vi "CCTestProgram.vi"() -> ()   [LabVIEW 2013, in "Medimatic.lvlib"]
uses:
  Medimatic.lvlib
  <userlib>/_MGI/Error Handling/MGI Suppress Error Code/MGI Suppress Error Code (Scalar).vi
  <vilib>/Utility/cursorutil.llb/Set Cursor (Icon Pict).vi
panel:
  out "patientsRetrieved":i32
  out "VerificationSCU":bool=TRUE
  in  "Exit":bool
  in  "queryWorklist":bool
  out "Worklist":string[][](array[string])
  in  "remotePort":i32=1234
  in  "remoteHost":string="localhost"
  in  "remoteAE":string="OFFIS"
  in  "clientAETitle":string="PseudoSCU"
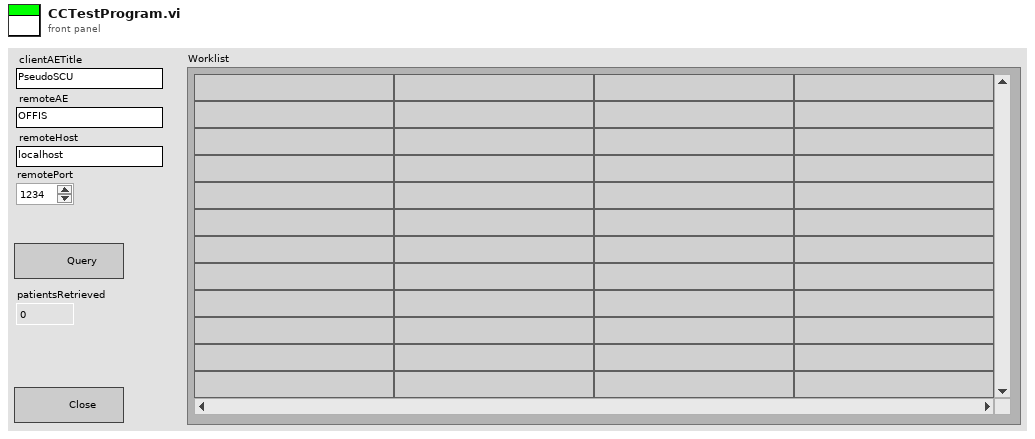
[diagram p1: front panel]
types:
  T1 = typedef "LVPoint32TypeDef.ctl" = cluster{"Horizontal":i32, "Vertical":i32}
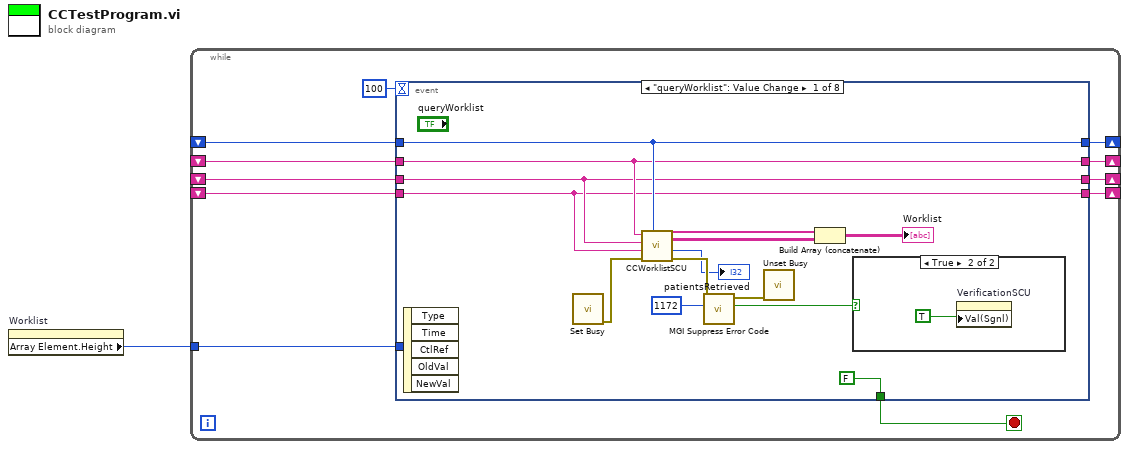
[diagram p0: block diagram]
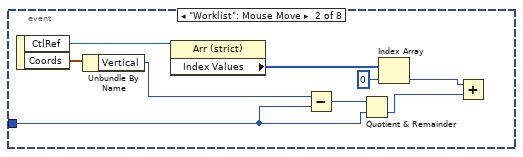
[diagram p3: hidden frame]
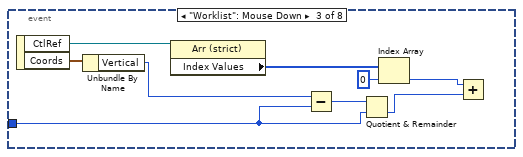
[diagram p4: hidden frame]
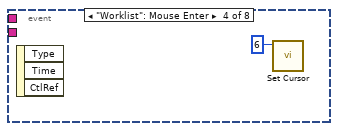
[diagram p5: hidden frame]
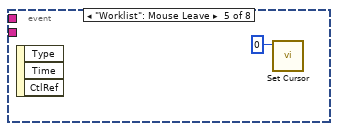
[diagram p6: hidden frame]
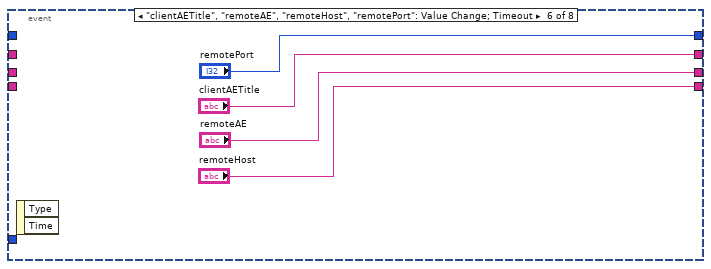
[diagram p7: hidden frame]
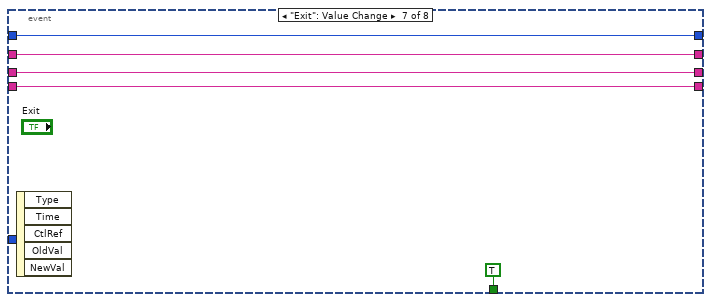
[diagram p8: hidden frame]
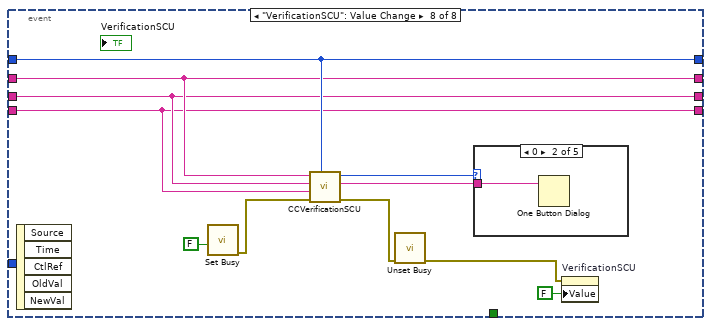
[diagram p9: hidden frame]
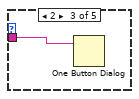
[diagram p11: hidden frame]
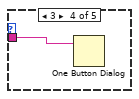
[diagram p12: hidden frame]
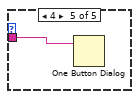
[diagram p13: hidden frame]
diagram:
  n1 = property on="Worklist" class="Arr (strict)"() -> ("Array Element.Height"=w1:u32)  [unwired: 2 in, 2 out]
  n2 = while {
    shift-right: [w11] -> _
    shift-left: _ -> [w7]
    shift-right: [w10] -> _
    shift-left: _ -> [w6]
    shift-right: [w9] -> _
    shift-left: _ -> [w5]
    shift-right: [w8] -> _
    shift-left: _ -> [w4]
    tunnel: w1 -> [w2]
    stop <- w12 stop-if-true
    n3 = event shown="[0] \"queryWorklist\": Value Change" {
      selector: _ -> [_ _ _ _ _ _ _ _]
      dyn-events: _ -> [_ _ _ _ _ _ _ _]
      timeout: 100 -> [_ _ _ _ _ _ _ _]
      tunnel: [FALSE _ _ _ _ _ TRUE _] -> w12
      tunnel: w4 -> [w18 _ _ _ _ _ w52 w59]
      tunnel: w5 -> [w19 _ _ _ _ _ w53 w60]
      tunnel: w6 -> [w20 _ _ _ _ _ w54 w61]
      tunnel: w7 -> [w21 _ _ _ _ _ w55 w62]
      tunnel: [w21 _ _ _ _ "remotePort" w55 w62] -> w11
      tunnel: [w20 _ _ _ _ "clientAETitle" w54 w61] -> w10
      tunnel: [w19 _ _ _ _ "remoteAE" w53 w60] -> w9
      tunnel: [w18 _ _ _ _ "remoteHost" w52 w59] -> w8
      tunnel: w2 -> [_ w30 w39 _ _ _ _ _]
      event "queryWorklist": Value Change {
        n4 = event-data() -> ()  [unwired: 1 in, 5 out]
        n5 = call <vilib>:"Set Busy.vi"() -> ("error out"=w17:errorcluster)  [unwired: 10 in, 1 out]
        n6 = call "CCWorklistSCU.vi"("remotePort"=w21, "error in (no error)"=w17, "remoteHost"=w18, "remoteAE"=w19, "clientAETitle"=w20) -> ("error out"=w16:errorcluster, "patientsRetrieved"=→"patientsRetrieved":i32, "Worklist"=w25:string[][], "DicomTags"=w26:string[])  [unwired: 2 in]
        n7 = call-poly <userlib>:"MGI Suppress Error Code.vi"("Error Code"=1172, "Error In"=w16) -> ("Error Supressed?"=w22:bool, "Error Out"=w15:errorcluster)  [unwired: 4 in]
        n8 = call <vilib>:"Unset Busy.vi"("error in (no error)"=w15) -> ()  [unwired: 10 in, 1 out]
        n9 = Build Array (concatenate)(w26, w25) -> (→"Worklist":string[][])
        n10 = case shown="True" w22 {
          frame False {
          }
          frame True {
            n11 = property on="VerificationSCU" class="Bool (strict)"("Val(Sgnl)"=TRUE) -> ()  [unwired: 2 in, 2 out]
          }
        }
      }
      event "Worklist": Mouse Move {
        n12 = event-data() -> ("CtlRef"=w36:refnum<vi>, "Coords"=w29:T1)  [unwired: 1 in]
        n13 = Unbundle By Name(w29) -> ("Vertical"=w28:i32)
        n14 = property class="Arr (strict)"(reference=w36) -> ("Index Values"=w35:u32[])  [unwired: 1 in, 2 out]
        n15 = Subtract(x=w28, y=w30) -> (x-y=w33:u32)
        n16 = Quotient & Remainder(x=w33, y=w30) -> (floor(x/y)=w31:u32)  [unwired: 1 out]
        n17 = Index Array(array=w35, index=0) -> (element=w32:u32)
        n18 = Add(x=w32, y=w31) -> ()  [unwired: 1 out]
      }
      event "Worklist": Mouse Down {
        n19 = event-data() -> ("CtlRef"=w45:refnum<vi>, "Coords"=w38:T1)  [unwired: 1 in]
        n20 = Unbundle By Name(w38) -> ("Vertical"=w37:i32)
        n21 = property class="Arr (strict)"(reference=w45) -> ("Index Values"=w44:u32[])  [unwired: 1 in, 2 out]
        n22 = Subtract(x=w37, y=w39) -> (x-y=w42:u32)
        n23 = Quotient & Remainder(x=w42, y=w39) -> (floor(x/y)=w40:u32)  [unwired: 1 out]
        n24 = Index Array(array=w44, index=0) -> (element=w41:u32)
        n25 = Add(x=w41, y=w40) -> ()  [unwired: 1 out]
      }
      event "Worklist": Mouse Enter {
        n26 = event-data() -> ()  [unwired: 1 in, 3 out]
        n27 = call-poly <vilib>:"Set Cursor.vi"("icon"=u16 6) -> ()  [unwired: 9 in, 2 out]
      }
      event "Worklist": Mouse Leave {
        n28 = event-data() -> ()  [unwired: 1 in, 3 out]
        n29 = call-poly <vilib>:"Set Cursor.vi"("icon"=u16 0) -> ()  [unwired: 9 in, 2 out]
      }
      event "clientAETitle", "remoteAE", "remoteHost", "remotePort": Value Change; Timeout {
        n30 = event-data() -> ()  [unwired: 1 in, 2 out]
      }
      event "Exit": Value Change {
        n31 = event-data() -> ()  [unwired: 1 in, 5 out]
      }
      event "VerificationSCU": Value Change {
        n32 = event-data() -> ()  [unwired: 1 in, 5 out]
        n33 = call <vilib>:"Set Busy.vi"("disable click? (T)"=FALSE) -> ("error out"=w65:errorcluster)  [unwired: 9 in, 1 out]
        n34 = call "CCVerificationSCU.vi"("remotePort"=w62, "error in (no error)"=w65, "remoteHost"=w59, "remoteAE"=w60, "clientAETitle"=w61) -> ("error out"=w64:errorcluster, "FailureDescription"=w66:string, "Result"=w67:i32)  [unwired: 4 in]
        n35 = call <vilib>:"Unset Busy.vi"("error in (no error)"=w64) -> ("error out"=w58:errorcluster)  [unwired: 10 in]
        n36 = case shown="0" w67 {
          tunnel: w66 -> [_ w68 w69 w70 w71]
          frame 1, Default {
          }
          frame 0 {
            n37 = One Button Dialog(message=w68) -> ()  [unwired: 1 in, 1 out]
          }
          frame 2 {
            n38 = One Button Dialog(message=w69) -> ()  [unwired: 1 in, 1 out]
          }
          frame 3 {
            n39 = One Button Dialog(message=w70) -> ()  [unwired: 1 in, 1 out]
          }
          frame 4 {
            n40 = One Button Dialog(message=w71) -> ()  [unwired: 1 in, 1 out]
          }
        }
        n41 = property on="VerificationSCU" class="Bool (strict)"(error in=w58, "Value"=FALSE ("Boolean")) -> ()  [unwired: 1 in, 2 out]
      }
    }
  }
